vi "Front Panel2_setup.vi"(1 "CHANNEL":bool, 2 "CONTROLLER TYPE":bool, 3 "GPIB Address":string) -> (0 "OK 2":bool)   [LabVIEW 2021]
uses:
  GL_DRCtype.vi
  GL_DRCchannel.vi
  GL_DRC_GPIBadd.vi
panel:
  in  "Cancel":bool
  in  "OK":bool
  # "e"
  # "e"
  # "TEMPERATURE \nREMOTE TEMPERATURE CONTROLLER"
  # "TEMPERATURE \nREMOTE TEMPERATURE CONTROLLER"
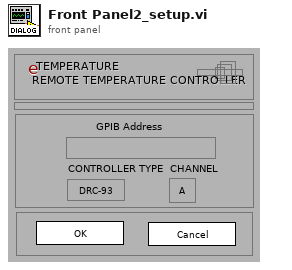
[diagram p1: front panel]
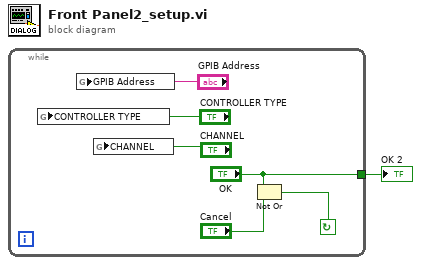
[diagram p0: block diagram]
diagram:
  n1 = while {
    tunnel: ["OK"] -> w1
    stop <- w7 continue-if-true
    n2 = global write "GL_DRCtype.vi" "CONTROLLER TYPE"("CONTROLLER TYPE") -> ()
    n3 = global write "GL_DRC_GPIBadd.vi" "GPIB Address"("GPIB Address") -> ()
    n4 = global write "GL_DRCchannel.vi" "CHANNEL"("CHANNEL") -> ()
    n5 = Not Or(1:"OK", 2:"Cancel") -> (0:w7:bool)
  }
  "OK 2" <- w1
